vi "Merge Error.vi"(10 "Error":errorcluster, 11 "Merge Error in":refnum<class "Merge Error.lvclass">) -> (3 "Merge Error out":refnum<class "Merge Error.lvclass">)   [LabVIEW 2021, in "Merge Error Msg Strategy.lvlib" / "Merge Error.lvclass"]
uses:
  Merge Error.lvclass
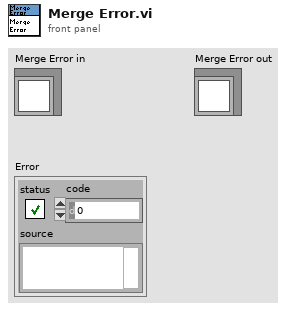
[diagram p1: front panel]
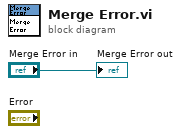
[diagram p0: block diagram]
diagram:
  "Merge Error out" <- "Merge Error in"
